vi "ExtractTypeFromFile.vi"(8 "error in (no error)":errorcluster, 10 "Type":string, 11 "Test in":refnum<class "Test.lvclass">) -> (0 "error out":errorcluster, 3 "PluginType":string)   [LabVIEW 2018]
doc: "This VI compares the input string labeld Type to the PluginType section in each ini file. If a match is found it returns the value found."
uses:
  NistPluggableModules/TestClass/Test.lvclass
  NistPluggableModules/TestClass/Test.lvclass/Test.ctl
  NistPluggableModules/TestClass/Accessors/Read PluginPathArray.vi
  <vilib>/Utility/config.llb/Read Key (String).vi
  <vilib>/Utility/error.llb/Error Cluster From Error Code.vi
  <vilib>/ErrorRing/Error Ring.xnode
  <vilib>/Utility/config.llb/NI_LVConfig.lvlib
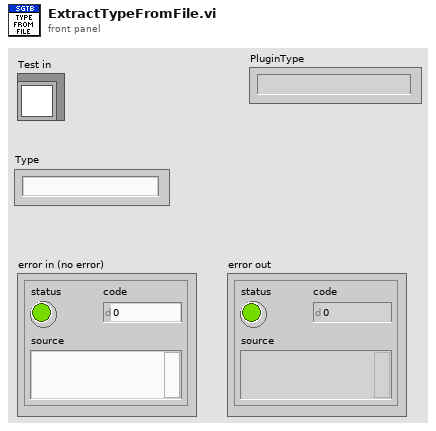
[diagram p1: front panel]
types:
  T1 = typedef "NI_LVConfig.lvlib/Config Data RefNum.ctl" = refnum<k1>
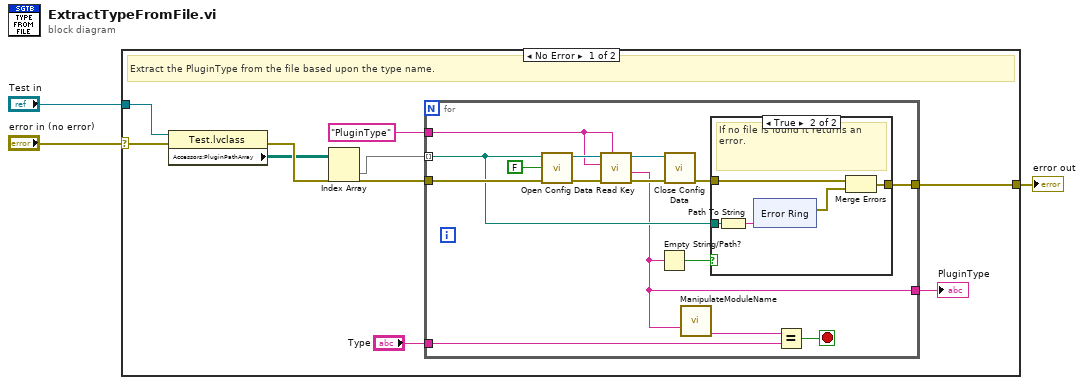
[diagram p0: block diagram]
diagram:
  n1 = case shown="No Error" "error in (no error)" {
    selector: "error in (no error)" -> [w11 w41]
    tunnel: "Test in" -> [w12 _]
    tunnel: [w8 w41] -> w1
    frame No Error {
      # "Extract the PluginType from the file based upon the type name."
      n2 = property class="Test.lvclass"(reference=w12, error in=w11) -> (error out=w10:errorcluster, "Accessors:PluginPathArray"=w6:path[][])  [unwired: 1 out]
      n3 = Index Array(array=w6) -> (element=w5:path[])  [unwired: 2 in]
      n4 = for {
        tunnel: w5 -> [w17] mode=indexing
        tunnel: "PluginType" ("section") -> [w20]
        tunnel: "Type" -> [w15]
        tunnel: [w19] -> w8
        tunnel: w10 -> [w18]
        tunnel: [w14] -> w7
        stop <- w16 stop-if-true
        n5 = call <vilib>:"Open Config Data.vi"("error in (no error)"=w18, "create file if necessary (T)"=FALSE, "configuration file path"=w17) -> ("error out"=w26:errorcluster, "refnum"=w25:T1)  [unwired: 6 in, 1 out]
        n6 = call-poly <vilib>:"Read Key.vi"("section"=w20, "error in (no error)"=w26, "key"=w20, "refnum"=w25) -> ("error out"=w23:errorcluster, "value"=w14:string, "refnum out"=w24:T1)  [unwired: 4 in, 1 out]
        n7 = Empty String/Path?(string/path=w14) -> (empty?=w22:bool)
        n8 = call <vilib>:"Close Config Data.vi"("error in (no error)"=w23, "refnum"=w24) -> ("error out"=w21:errorcluster)  [unwired: 8 in, 1 out]
        n9 = call "ManipulateModuleName.vi"("ModuleListSingleEntry"=w14) -> ("AfterMatch:ModuleListSingleEntry"=w13:string)  [unwired: 9 in, 5 out]
        n10 = case shown="True" w22 {
          tunnel: w21 -> [w28 w32]
          tunnel: [w28 w31] -> w19
          tunnel: w17 -> [_ w29]
          frame False {
          }
          frame True {
            # "If no file is found it returns an error."
            n11 = Path To String(path=w29) -> (string=w30:string)
            n12 = xnode "Error Ring"("parameter 0"=w30) -> ("error out"=w33:errorcluster)
            n13 = Merge Errors(w32, w33) -> (w31:errorcluster)
          }
        }
        n14 = Equal?(x=w13, y=w15) -> (x = y?=w16:bool)
      }
      "PluginType" <- w7
    }
    frame Error {
    }
  }
  "error out" <- w1
